vi "SetParam.vi"(8 "error in (no error)":errorcluster caption="entrée d'erreur (pas d'erreur)", 10 "matthews_corrcoef":cluster{"sample_weight":dbl[]}, 11 "Matthews_Corrcoef.lvclass":refnum<class "Matthews_Corrcoef.lvclass">) -> (0 "error out":errorcluster caption="sortie d'erreur", 3 "Matthews_Corrcoef.lvclass":refnum<class "Matthews_Corrcoef.lvclass">)   [LabVIEW 2020, in "Matthews_Corrcoef.lvclass"]
doc: "Set Parameters"
uses:
  Matthews_Corrcoef.lvclass
  Matthews_Corrcoef.lvclass/Matthews_Corrcoef.ctl
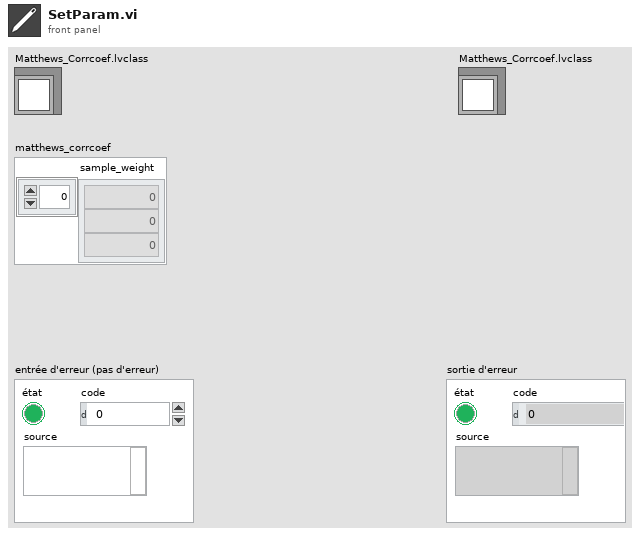
[diagram p1: front panel]
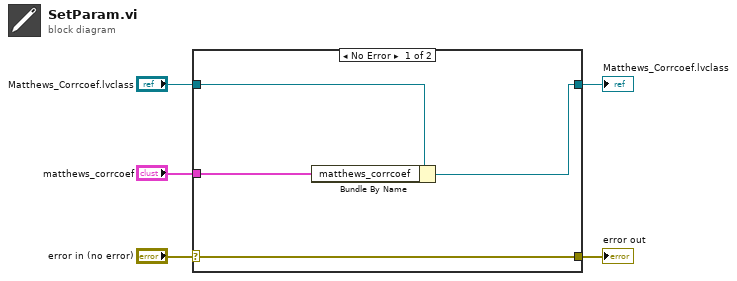
[diagram p0: block diagram]
diagram:
  n1 = case shown="No Error" "error in (no error)" {
    selector: "error in (no error)" -> [w9 w10]
    tunnel: [w9 w10] -> w4
    tunnel: [w7 w11] -> w2
    tunnel: "Matthews_Corrcoef.lvclass" -> [w8 w11]
    tunnel: "matthews_corrcoef" -> [w6 _]
    frame No Error {
      n2 = Bundle By Name(cluster=w8, "matthews_corrcoef"=w6) -> (w7:refnum<class "Matthews_Corrcoef.lvclass">)
    }
    frame Error {
    }
  }
  "error out" <- w4
  "Matthews_Corrcoef.lvclass" <- w2
